vi "Exponents--contant.vi"() -> (1 "exponent":dbl[](array[numeric])=[-2.0, -1.0, 0.0, 0.0, 1.0, 2.0, 3.0, 4.0, 5.0, 6.0, 7.0, 8.0, 9.0])   [LabVIEW 2018, in "Resistance Values.lvlib"]
uses:
  Resistance Values.lvlib
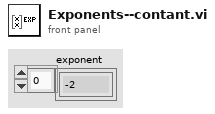
[diagram p1: front panel]
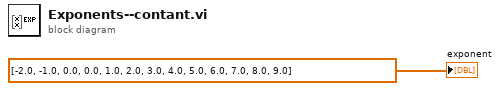
[diagram p0: block diagram]
diagram:
  "exponent" <- dbl[] [-2.0, -1.0, 0.0, 0.0, 1.0, 2.0, 3.0, 4.0, 5.0, 6.0, 7.0, 8.0, 9.0]
